vi "AutonCals.vi"() -> ()   [LabVIEW 2014]
panel:
  in  "RotationEpsilon":dbl=3.0
  in  "RotationD":dbl=0.01
  in  "RotationI":dbl=0.01
  in  "RotationP":dbl=0.028
  in  "SpeedEpsilon":dbl=0.1
  in  "DistanceEpsilon":dbl=0.5
  in  "StrafeD":dbl=0.05
  in  "StrafeI":dbl
  in  "StrafeP":dbl=2.0
  in  "DriveD":dbl=0.001
  in  "DriveI":dbl=0.03
  in  "DriveP":dbl=0.48
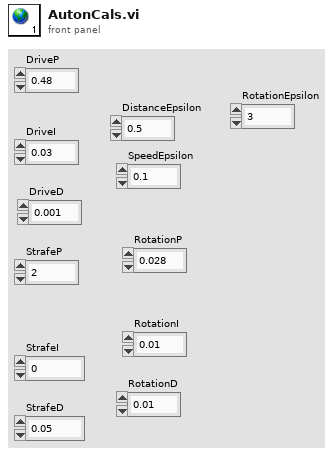
[diagram p1: front panel]
diagram:
